vi "Scan Engine Generic IOV Channel Page.vi"(8 "error in (no error)":errorcluster, 11 "Node Ptr":T1 format="%.0x") -> (0 "error out":errorcluster)   [LabVIEW 2020, in "SEECD System Explorer.lvlib"]
uses:
  SEECD System Explorer.lvlib
  <vilib>/NI VeriStand/Custom Device API/Custom Device Item Ref.ctl
  <vilib>/NI VeriStand/Custom Device API/Custom Device Channel Type.ctl
  <vilib>/NI VeriStand/Custom Device API/Custom Device API.lvlib
panel:
  out "Channel Settings":i32(listbox)
  in  "Default Value":dbl
  in  "Header":cluster{"Section Name":string}={"Section Name"="Hardware IO Item Settings"}
  in  "Description":string
  in  "Name":string
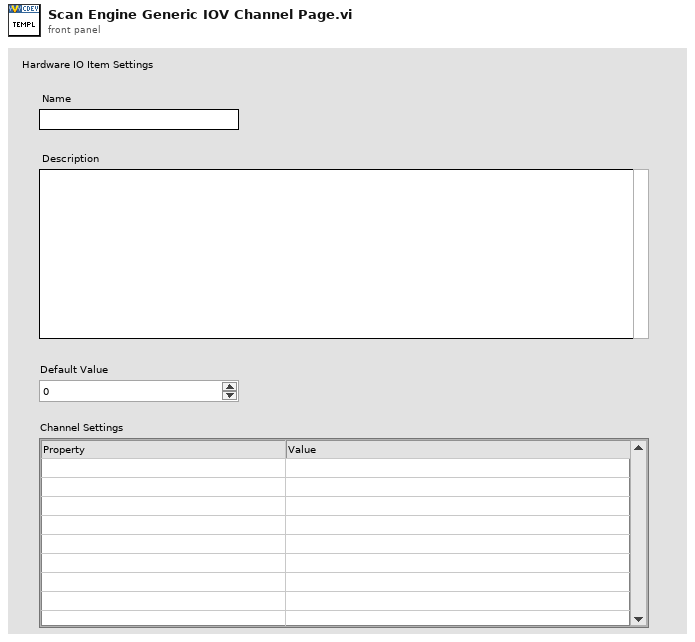
[diagram p1: front panel]
types:
  T1 = typedef "Custom Device API.lvlib/Custom Device Item Ref.ctl" = u64
  T2 = typedef "Custom Device API.lvlib/Custom Device Channel Type.ctl" = enum16{"Input", "Output"}
  T3 = typedef "Custom Device API.lvlib/Custom Device Item Info.ctl" = cluster{"Name":string, "Is Channel":bool, "GUID":string, "Is Waveform":bool}
  T4 = typedef "Custom Device API.lvlib/Custom Device Channel.ctl" = cluster{"Type":T2, "Units":string, "Default Value":dbl, "Faultable":bool, "Scalable":bool}
  T5 = typedef "Custom Device API.lvlib/Custom Device Commands.ctl" = enum16{"Default", "Item renamed", "Shutdown", "Dynamic button pressed"}
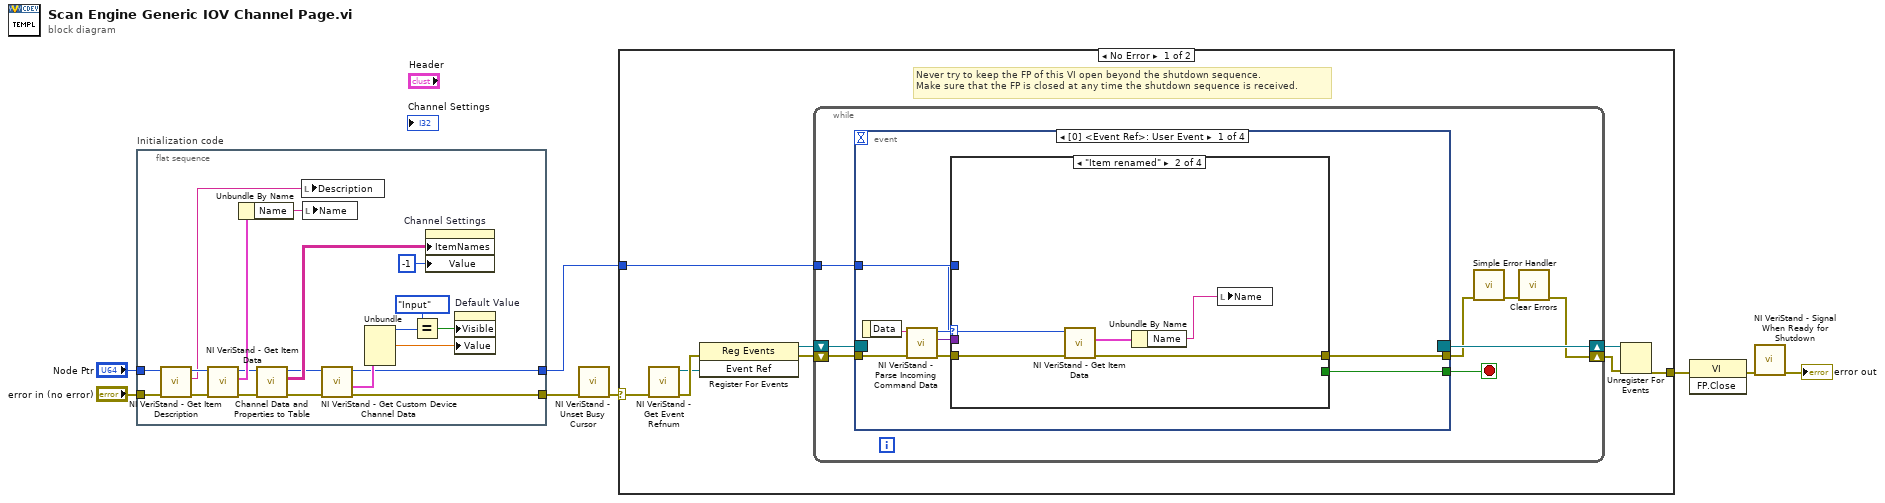
[diagram p0: block diagram]
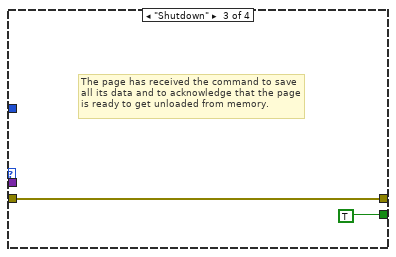
[diagram p3: hidden frame]
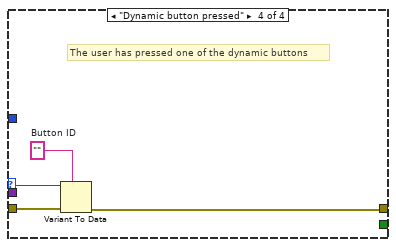
[diagram p4: hidden frame]
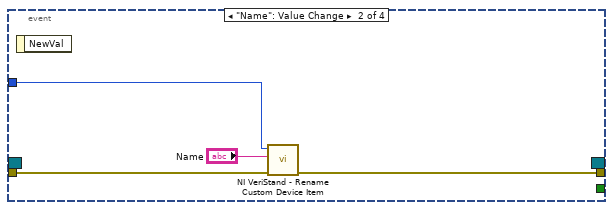
[diagram p5: hidden frame]
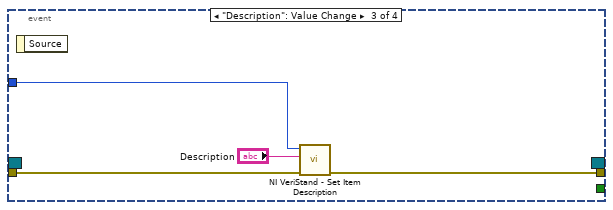
[diagram p6: hidden frame]
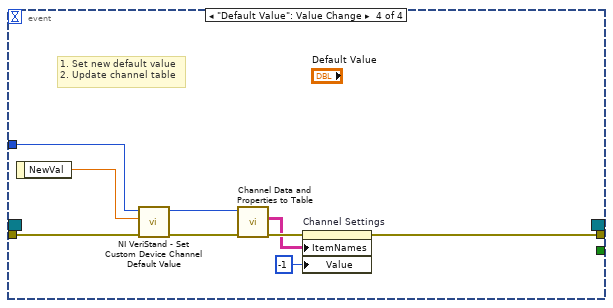
[diagram p7: hidden frame]
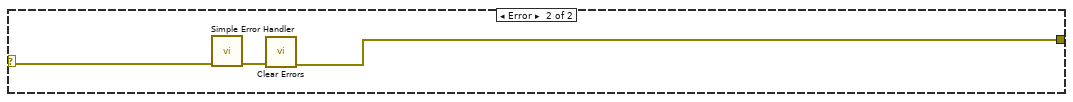
[diagram p8: hidden frame]
diagram:
  n1 = flat-sequence "Initialization code" {
    tunnel: "error in (no error)" -> [w27]
    tunnel: "Node Ptr" -> [w26]
    tunnel: [w9] -> w4
    tunnel: [w10] -> w1
    frame #0 {
      n2 = call <vilib>:"NI VeriStand - Get Item Description.vi"("error in (no error)"=w27, "Item Ref in"=w26) -> ("error out"=w24:errorcluster, "Description"=w25:string, "Item Ref out"=w28:T1)  [unwired: 7 out]
      n3 = call <vilib>:"NI VeriStand - Get Item Data.vi"("error in (no error)"=w24, "Item Ref in"=w28) -> ("error out"=w20:errorcluster, "Item Info"=w23:T3, "Item Ref out"=w21:T1)  [unwired: 7 out]
      n4 = Unbundle By Name(w23) -> ("Name"=w22:string)
      n5 = call "Channel Data and Properties to Table.vi"("error in (no error)"=w20, "Node Ptr"=w21) -> ("error out"=w11:errorcluster, "Properties List Out"=w18:string[][], "Channel Ref out"=w12:T1)  [unwired: 7 in]
      n6 = local write "Description"(w25) -> ()
      n7 = local write "Name"(w22) -> ()
      n8 = call <vilib>:"NI VeriStand - Get Custom Device Channel Data.vi"("error in (no error)"=w11, "Channel Ref in"=w12) -> ("error out"=w9:errorcluster, "Channel"=w14:T4, "Channel Ref out"=w10:T1)  [unwired: 4 in, 3 out]
      n9 = Unbundle(w14) -> ("Type"=w16:T2, "Default Value"=w17:dbl)  [unwired: 3 out]
      n10 = Equal?(x=Custom_Device_Channel_Type."Input" ("Type"), y=w16) -> (x = y?=w15:bool)
      n11 = property on="Channel Settings" class="MCListbox (strict)"("ItemNames"=w18, "Value"=-1 ("Channel Settings")) -> ()  [unwired: 2 in, 2 out]
      n12 = property on="Default Value" class="DigNum (strict)"("Visible"=w15, "Value"=w17) -> ()  [unwired: 2 in, 2 out]
    }
  }
  n13 = call <vilib>:"NI VeriStand - Unset Busy Cursor.vi"("error in (no error)"=w4) -> ("error out"=w3:errorcluster)  [unwired: 10 out]
  n14 = case shown="No Error" w3 {
    selector: w3 -> [w29 w85]
    tunnel: [w34 w83] -> w8
    tunnel: w1 -> [w30 _]
    frame No Error {
      # "Never try to keep the FP of this VI open beyond the shutdown sequence.\nMake sure that the FP is closed at any time the shutdown sequence is received."
      n15 = call <vilib>:"NI VeriStand - Get Event Refnum.vi"("error in (no error)"=w29) -> ("error out"=w37:errorcluster, "Event Ref"=w33:refnum<user-event>)  [unwired: 9 out]
      n16 = register-events(error in=w37, w33) -> (reference out=w31:refnum<event-registration>, error out=w32:errorcluster)  [unwired: 1 in]
      n17 = while {
        tunnel: w30 -> [w41]
        shift-right: [w38] -> w35
        shift-left: w32 -> [w44]
        shift-right: [w45] -> w36
        shift-left: w31 -> [w43]
        stop <- w42 stop-if-true
        n18 = event shown="[0] <Event Ref>: User Event" {
          selector: w43 -> [_ _ _ _]
          dyn-events: [_ _ _ _] -> w45
          timeout: _ -> [_ _ _ _]
          tunnel: w44 -> [w53 w69 w72 w80]
          tunnel: [w49 _ _ _] -> w42
          tunnel: [w48 w68 w71 w76] -> w40
          tunnel: w41 -> [w47 w67 w73 w81]
          event User Event {
            n19 = event-data() -> ("Data"=w52:string)  [unwired: 1 out]
            n20 = call <vilib>:"NI VeriStand - Parse Incoming Command Data.vi"("error in (no error)"=w53, "Incoming data"=w52) -> ("error out"=w51:errorcluster, "Outgoing data"=w46:variant, "Action"=w50:T5)  [unwired: 7 out]
            n21 = case shown="\"Item renamed\"" w50 {
              tunnel: w51 -> [w54 w59 w60 w65]
              tunnel: [_ _ TRUE _] -> w49
              tunnel: [w54 w56 w60 w62] -> w48
              tunnel: w47 -> [_ w58 _ _]
              tunnel: w46 -> [_ _ _ w64]
              frame "Default", Default {
              }
              frame "Item renamed" {
                n22 = call <vilib>:"NI VeriStand - Get Item Data.vi"("error in (no error)"=w59, "Item Ref in"=w58) -> ("error out"=w56:errorcluster, "Item Info"=w57:T3)  [unwired: 8 out]
                n23 = Unbundle By Name(w57) -> ("Name"=w55:string)
                n24 = local write "Name"(w55) -> ()
              }
              frame "Shutdown" {
                # "The page has received the command to save all its data and to acknowledge that the page is ready to get unloaded from memory."
              }
              frame "Dynamic button pressed" {
                w63 = ""  # Button ID
                # "The user has pressed one of the dynamic buttons"
                n25 = Variant To Data(error in=w65, type=w63, Variant=w64) -> (error out=w62:errorcluster)  [unwired: 1 out]
              }
            }
          }
          event "Name": Value Change {
            n26 = event-data() -> ()  [unwired: 2 out]
            n27 = call <vilib>:"NI VeriStand - Rename Custom Device Item.vi"("error in (no error)"=w69, "New Name"="Name", "Item Ref in"=w67) -> ("error out"=w68:errorcluster)  [unwired: 1 in, 7 out]
          }
          event "Description": Value Change {
            n28 = event-data() -> ()  [unwired: 2 out]
            n29 = call <vilib>:"NI VeriStand - Set Item Description.vi"("error in (no error)"=w72, "Description"="Description", "Item Ref in"=w73) -> ("error out"=w71:errorcluster)  [unwired: 8 out]
          }
          event "Default Value": Value Change {
            # "1. Set new default value\n2. Update channel table"
            n30 = event-data() -> ("NewVal"=w82:dbl)  [unwired: 1 out]
            n31 = call <vilib>:"NI VeriStand - Set Custom Device Channel Default Value.vi"("error in (no error)"=w80, "Default Value"=w82, "Channel Ref in"=w81) -> ("error out"=w78:errorcluster, "Channel Ref out"=w74:T1)  [unwired: 7 in]
            n32 = call "Channel Data and Properties to Table.vi"("error in (no error)"=w78, "Node Ptr"=w74) -> ("error out"=w77:errorcluster, "Properties List Out"=w75:string[][])  [unwired: 7 in, 1 out]
            n33 = property on="Channel Settings" class="MCListbox (strict)"(error in=w77, "ItemNames"=w75, "Value"=-1 ("Channel Settings")) -> (error out=w76:errorcluster)  [unwired: 1 in, 1 out]
          }
        }
        n34 = call <vilib>:"Simple Error Handler.vi"("error in (no error)"=w40) -> ("error out"=w39:errorcluster)  [unwired: 1 in, 7 out]
        n35 = call <vilib>:"Clear Errors.vi"("error in (no error)"=w39) -> ("error out"=w38:errorcluster)  [unwired: 1 in, 5 out]
      }
      n36 = Unregister For Events(event registration refnum=w36, error in=w35) -> (error out=w34:errorcluster)
    }
    frame Error {
      n37 = call <vilib>:"Simple Error Handler.vi"("error in (no error)"=w85) -> ("error out"=w84:errorcluster)  [unwired: 1 in, 7 out]
      n38 = call <vilib>:"Clear Errors.vi"("error in (no error)"=w84) -> ("error out"=w83:errorcluster)  [unwired: 1 in, 5 out]
    }
  }
  n39 = invoke class="VI" method="FP.Close"(error in=w8) -> (error out=w7:errorcluster)  [unwired: 2 in, 2 out]
  n40 = call <vilib>:"NI VeriStand - Signal When Ready for Shutdown.vi"("error in (no error)"=w7) -> ("error out"=→"error out":errorcluster)  [unwired: 10 out]
